vi "Module.Default Tasks2.vi"(7 "Sys":T1, 8 "error in":errorcluster, 9 "Data2":variant, 10 "Data1":variant, 11 "Sub":string) -> (0 "error out":errorcluster, 5 "Sys Out":T1)   [LabVIEW 2024, in "EQMF.lvlib" / "Module Utils.lvlib"]
uses:
  Module Utils.lvlib
  Module Sys Info.ctl
  Config/Stored Controls/Class.SaveCtrls.lvclass
  Event Log/Event Notification/Event Notification.lvclass
  Config/App Data/Class.AppData.lvclass
  Subscription/Subscription.lvclass
  Queues/Q.Element.ctl
  Module.SW Version Info.ctl
  Module Config.ctl
  Module.Working Dirs.ctl
  Event Log/Event Notification/Event Log.Log Level.ctl
  Menu/Menu Utils.lvlib
  Config/Config Utils.lvlib
  Queues/Queue Utils.lvlib
  Event Log/Event Log.lvlib
panel:
  # "Name, PN, Version, Note"
  # "Name, PN, Version, Note"
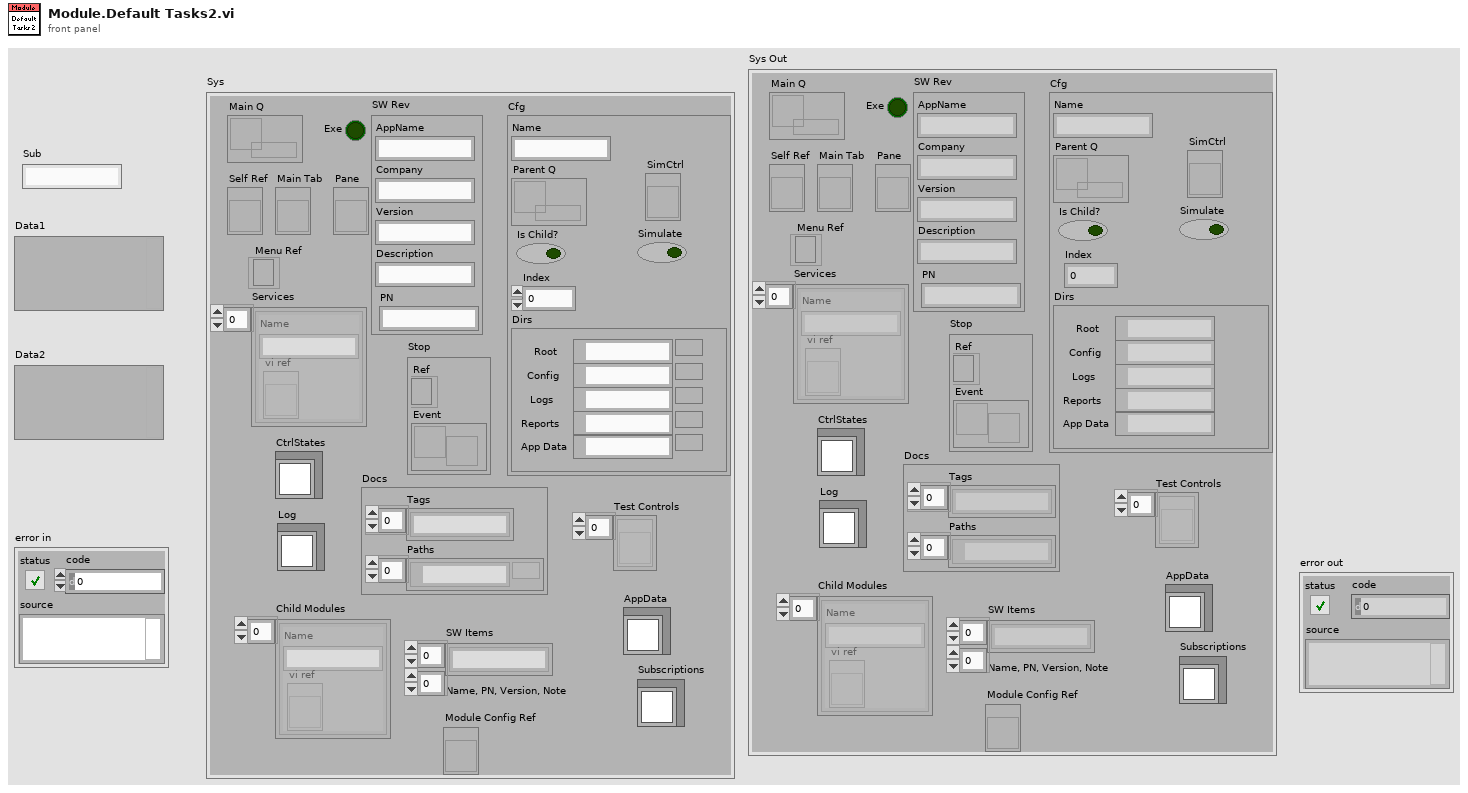
[diagram p1: front panel]
types:
  T1 = typedef "EQMF.lvlib/Module Utils.lvlib/Module Sys Info.ctl" = cluster{"Main Q":refnum<queue>, "Exe":bool, "SW Rev":T2, "Self Ref":refnum<vi>, "Main Tab":refnum<vi>, "Pane":refnum<vi>, "Stop":cluster{"Ref":refnum<event-registration>, "Event":refnum<user-event>}, "Cfg":T3, "Services":cluster{"Name":string, "vi ref":refnum<vi>}[], "Menu Ref":refnum<k9>, "CtrlStates":refnum<class "Class.SaveCtrls.lvclass">, "Docs":cluster{"Tags":string[], "Paths":path[]}, "Log":refnum<class "Event Notification.lvclass">, "Test Controls":refnum<vi>[], "Child Modules":cluster{"Name":string, "vi ref":refnum<vi>}[], "SW Items":string[][], "AppData":refnum<class "Class.AppData.lvclass">, "Subscriptions":refnum<class "Subscription.lvclass">, "Module Config Ref":refnum<vi>}
  T2 = typedef "EQMF.lvlib/Module Utils.lvlib/Module.SW Version Info.ctl" = cluster{"AppName":string, "Company":string, "Version":string, "Description":string, "PN":string}
  T3 = typedef "EQMF.lvlib/Module Utils.lvlib/Module Config.ctl" = cluster{"Name":string, "Parent Q":refnum<queue>, "Is Child?":bool, "Index":i32, "Dirs":T4, "Simulate":bool, "SimCtrl":refnum<vi>}
  T4 = typedef "EQMF.lvlib/Module Utils.lvlib/Module.Working Dirs.ctl" = cluster{"Root":path, "Config":path, "Logs":path, "Reports":path, "App Data":path}
  T5 = typedef "EQMF.lvlib/Event Log.lvlib/Event Log.Log Level.ctl" = enum16{"Normal", "Verbose", "Debug0", "Debug1", "Debug2"}
  T6 = enum8{"Enabled", "Disabled", "Disabled and Grayed Out"}
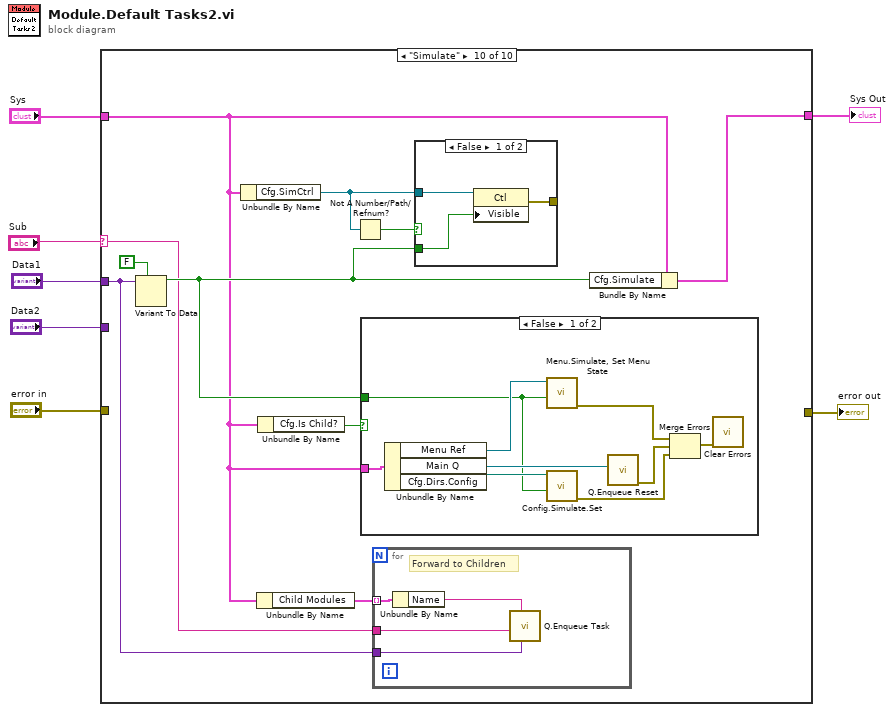
[diagram p0: block diagram]
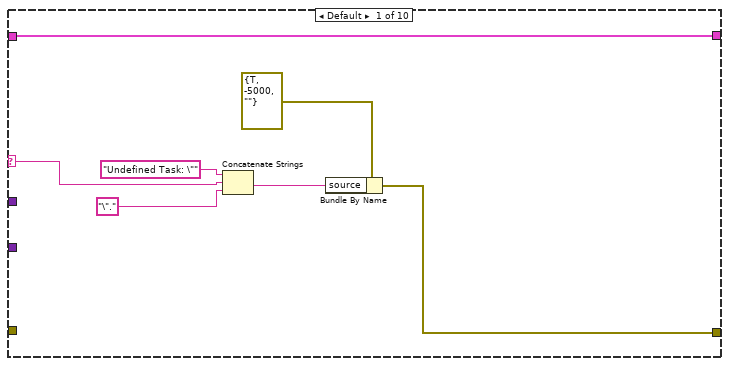
[diagram p2: hidden frame]
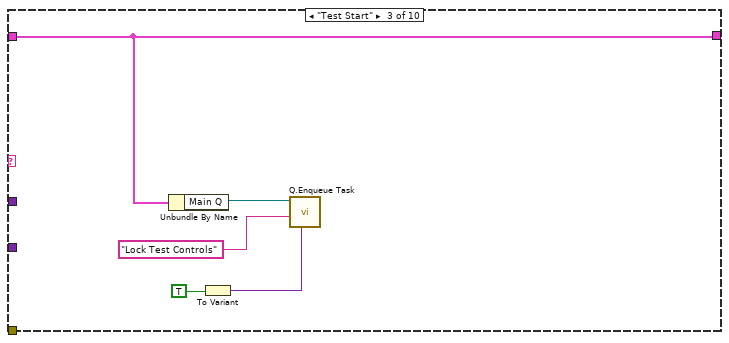
[diagram p4: hidden frame]
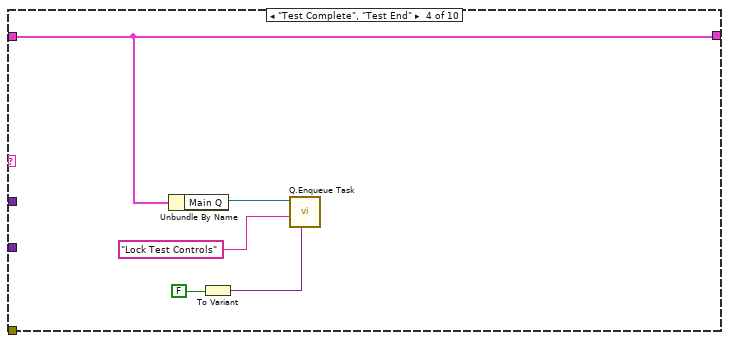
[diagram p5: hidden frame]
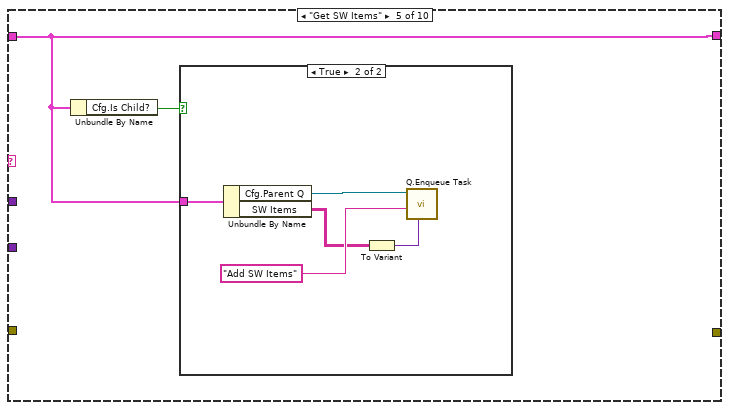
[diagram p6: hidden frame]
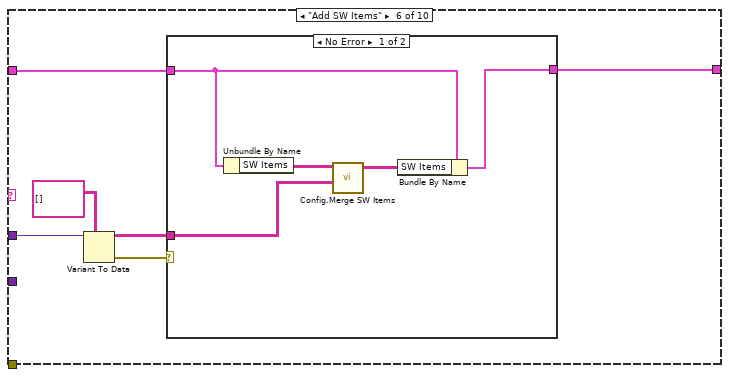
[diagram p8: hidden frame]
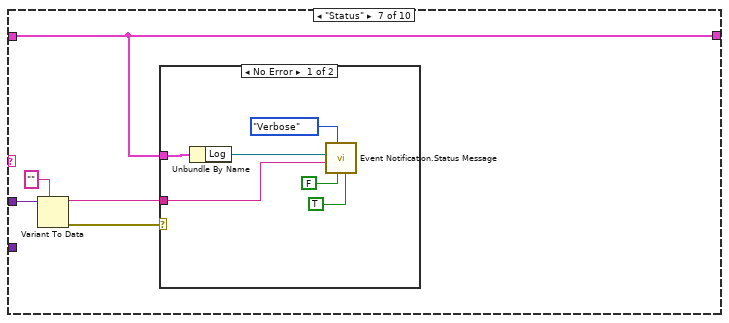
[diagram p10: hidden frame]
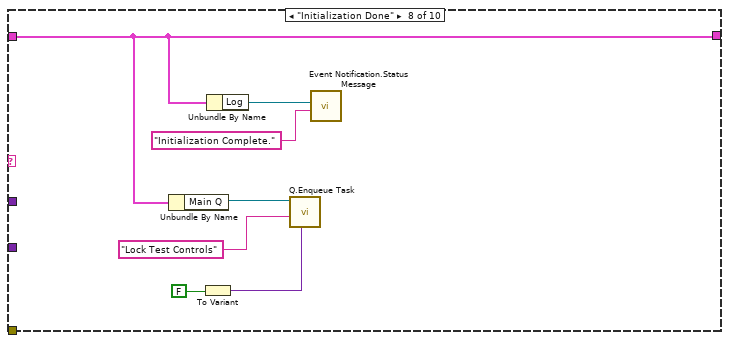
[diagram p12: hidden frame]
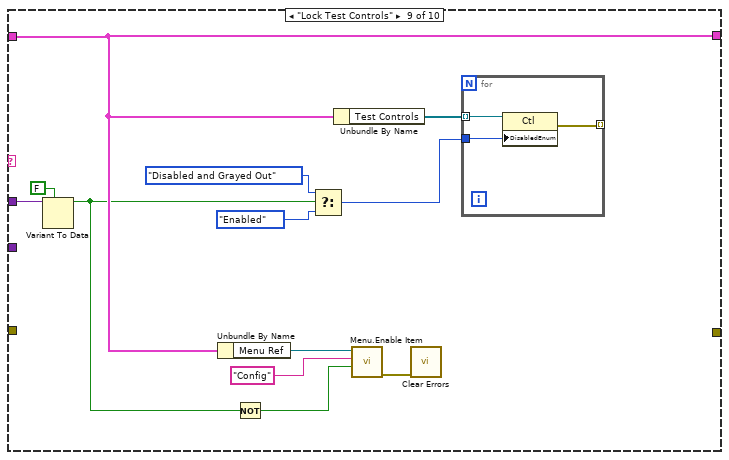
[diagram p13: hidden frame]
diagram:
  n1 = case shown="\"Simulate\"" "Sub" {
    selector: "Sub" -> [w12 _ _ _ _ _ _ _ _ w79]
    tunnel: "Sys" -> [w8 w15 w20 w21 w27 w34 w49 w58 w68 w81]
    tunnel: "Data1" -> [_ _ _ _ _ w38 w48 _ w72 w78]
    tunnel: "Data2" -> [_ _ _ _ _ _ _ _ _ _]
    tunnel: "error in" -> [_ _ _ _ _ _ _ _ _ _]
    tunnel: [w10 _ _ _ _ _ _ _ _ _] -> w2
    tunnel: [w8 w15 w20 w21 w27 w36 w49 w58 w68 w84] -> w1
    frame Default {
      n2 = Concatenate Strings("Undefined Task: \"", w12, "\".") -> (w9:string)
      n3 = Bundle By Name(cluster=errorcluster {"status"=TRUE, "code"=-5000, "source"=""} ("error constant"), "source"=w9) -> (w10:errorcluster)
    }
    frame "Test Abort", "Test Reset" {
      # "If this case is reached then the Task case statement does not have its own case.\nDo Nothing"
    }
    frame "Test Start" {
      n4 = Unbundle By Name(w20) -> ("Main Q"=w19:refnum<queue>)
      n5 = To Variant(anything=TRUE) -> (Variant=w17:variant)
      n6 = call "Q.Enqueue Task.vi"("Data1"=w17, "Task Name"="Lock Test Controls", "Q In"=w19) -> ()  [unwired: 7 in, 2 out]
    }
    frame "Test Complete", "Test End" {
      n7 = Unbundle By Name(w21) -> ("Main Q"=w25:refnum<queue>)
      n8 = To Variant(anything=FALSE) -> (Variant=w23:variant)
      n9 = call "Q.Enqueue Task.vi"("Data1"=w23, "Task Name"="Lock Test Controls", "Q In"=w25) -> ()  [unwired: 7 in, 2 out]
    }
    frame "Get SW Items" {
      n10 = Unbundle By Name(w27) -> ("Cfg.Is Child?"=w26:bool)
      n11 = case shown="True" w26 {
        tunnel: w27 -> [_ w32]
        frame False {
        }
        frame True {
          n12 = Unbundle By Name(w32) -> ("Cfg.Parent Q"=w31:refnum<queue>, "SW Items"=w29:string[][])
          n13 = To Variant(anything=w29) -> (Variant=w28:variant)
          n14 = call "Q.Enqueue Task.vi"("Data1"=w28, "Task Name"="Add SW Items", "Q In"=w31) -> ()  [unwired: 7 in, 2 out]
        }
      }
    }
    frame "Add SW Items" {
      n15 = Variant To Data(type=string[][] [], Variant=w38) -> (data=w35:string[][], error out=w33:errorcluster)  [unwired: 1 in]
      n16 = case shown="No Error" w33 {
        tunnel: [w41 w44] -> w36
        tunnel: w35 -> [w40 _]
        tunnel: w34 -> [w39 w44]
        frame No Error {
          n17 = Unbundle By Name(w39) -> ("SW Items"=w43:string[][])
          n18 = call "Config.Merge SW Items.vi"("SW Items"=w40, "SW List In"=w43) -> ("SW List Out"=w42:string[][])  [unwired: 8 in, 1 out]
          n19 = Bundle By Name(cluster=w39, "SW Items"=w42) -> (w41:T1)
        }
        frame Error {
        }
      }
    }
    frame "Status" {
      n20 = Variant To Data(type="", Variant=w48) -> (data=w46:string, error out=w45:errorcluster)  [unwired: 1 in]
      n21 = case shown="No Error" w45 {
        tunnel: w49 -> [w55 _]
        tunnel: w46 -> [w50 _]
        frame No Error {
          n22 = Unbundle By Name(w55) -> ("Log"=w54:refnum<class "Event Notification.lvclass">)
          n23 = call "Event Notification.Status Message.vi"("Display"=TRUE, "Log"=FALSE, "Level"=Event_Log.Log_Level."Verbose", "Message"=w50, "Event Notification in"=w54) -> ()  [unwired: 7 in]
        }
        frame Error {
        }
      }
    }
    frame "Initialization Done" {
      n24 = Unbundle By Name(w58) -> ("Main Q"=w62:refnum<queue>)
      n25 = To Variant(anything=FALSE) -> (Variant=w60:variant)
      n26 = Unbundle By Name(w58) -> ("Log"=w57:refnum<class "Event Notification.lvclass">)
      n27 = call "Q.Enqueue Task.vi"("Data1"=w60, "Task Name"="Lock Test Controls", "Q In"=w62) -> ()  [unwired: 7 in, 2 out]
      n28 = call "Event Notification.Status Message.vi"("Message"="Initialization Complete.", "Event Notification in"=w57) -> ()  [unwired: 10 in]
    }
    frame "Lock Test Controls" {
      n29 = Variant To Data(type=FALSE, Variant=w72) -> (data=w65:bool)  [unwired: 1 in, 1 out]
      n30 = Unbundle By Name(w68) -> ("Menu Ref"=w67:refnum<k9>)
      n31 = Not(x=w65) -> (.not. x?=w64:bool)
      n32 = Select(t=T6."Disabled and Grayed Out" ("Disabled"), s=w65, f=T6."Enabled" ("Disabled")) -> (s? t:f=w73:T6)
      n33 = Unbundle By Name(w68) -> ("Test Controls"=w74:refnum<vi>[])
      n34 = call "Menu.Enable Item.vi"("Enable"=w64, "Tag"="Config", "Menu Ref"=w67) -> ("error out"=w63:errorcluster)  [unwired: 7 in, 1 out]
      n35 = call <vilib>:"Clear Errors.vi"("error in (no error)"=w63) -> ()  [unwired: 5 in, 2 out]
      n36 = for {
        tunnel: w74 -> [w77] mode=indexing
        tunnel: w73 -> [w76]
        tunnel: [w75] -> _ mode=indexing
        n37 = property class="Ctl"(reference=w77, "DisabledEnum"=w76) -> (error out=w75:errorcluster)  [unwired: 1 in, 1 out]
      }
    }
    frame "Simulate" {
      n38 = Variant To Data(type=FALSE, Variant=w78) -> (data=w83:bool)  [unwired: 1 in, 1 out]
      n39 = Unbundle By Name(w81) -> ("Cfg.SimCtrl"=w86:refnum<vi>)
      n40 = Unbundle By Name(w81) -> ("Child Modules"=w80:cluster{"Name":string, "vi ref":refnum<vi>}[])
      n41 = Unbundle By Name(w81) -> ("Cfg.Is Child?"=w82:bool)
      n42 = Not A Number/Path/Refnum?(number/path/refnum=w86) -> (NaN/Path/Refnum?=w85:bool)
      n43 = case shown="False" w82 {
        tunnel: w81 -> [w100 _]
        tunnel: w83 -> [w96 _]
        frame False {
          n44 = Unbundle By Name(w100) -> ("Menu Ref"=w97:refnum<k9>, "Main Q"=w98:refnum<queue>, "Cfg.Dirs.Config"=w99:path)
          n45 = call "Menu.Simulate, Set Menu State.vi"("Sim Enable"=w96, "Menu Ref"=w97) -> ("error out"=w93:errorcluster)  [unwired: 8 in, 1 out]
          n46 = call "Config.Simulate.Set.vi"("Simulate"=w96, "Config Folder"=w99) -> ("error out"=w95:errorcluster)  [unwired: 9 in]
          n47 = call "Q.Enqueue Reset.vi"("Q In"=w98) -> ("error out"=w94:errorcluster)  [unwired: 9 in, 1 out]
          n48 = Merge Errors(w93, w94, w95) -> (w92:errorcluster)
          n49 = call <vilib>:"Clear Errors.vi"("error in (no error)"=w92) -> ()  [unwired: 5 in, 2 out]
        }
        frame True {
        }
      }
      n50 = for {
        tunnel: w80 -> [w91] mode=indexing
        tunnel: w79 -> [w89]
        tunnel: w78 -> [w88]
        # "Forward to Children"
        n51 = Unbundle By Name(w91) -> ("Name"=w90:string)
        n52 = call "Q.Enqueue Task.vi"("Data1"=w88, "Q Name"=w90, "Task Name"=w89) -> ()  [unwired: 7 in, 2 out]
      }
      n53 = case shown="False" w85 {
        tunnel: w86 -> [w103 _]
        tunnel: [w102 _] -> _
        tunnel: w83 -> [w101 _]
        frame False {
          n54 = property class="Ctl"(reference=w103, "Visible"=w101) -> (error out=w102:errorcluster)  [unwired: 1 in, 1 out]
        }
        frame True {
        }
      }
      n55 = Bundle By Name(cluster=w81, "Cfg.Simulate"=w83) -> (w84:T1)
    }
  }
  "error out" <- w2
  "Sys Out" <- w1
